vi "S-Curve Newton Method Time.vi"(4 "v_f":dbl, 6 "v_i":dbl, 7 "err":dbl, 8 "g":dbl, 9 "j":dbl, 10 "a":dbl, 11 "v":dbl) -> (3 "t_out":dbl)   [LabVIEW 2025]
uses:
  <vilib>/ptbypt/NI_PtbyPt.lvlib
panel:
  out "iterations":i32
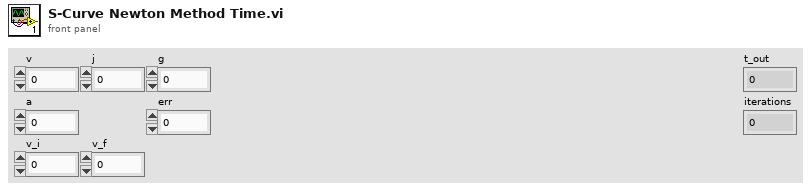
[diagram p1: front panel]
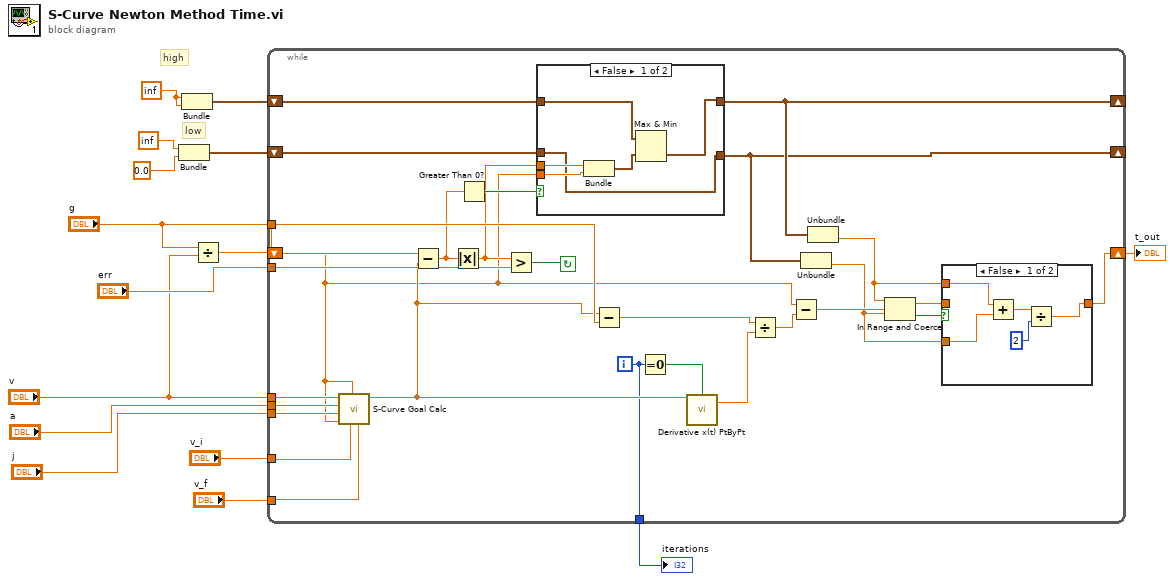
[diagram p0: block diagram]
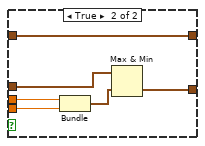
[diagram p2: hidden frame]
diagram:
  w6 = inf
  # "low"
  # "high"
  n1 = Bundle(inf, 0.0) -> (w2:cluster{dbl, dbl})  [unwired: 1 in]
  n2 = Bundle(w6, w6) -> (w5:cluster{dbl, dbl})  [unwired: 1 in]
  n3 = Divide(x="g", y="v") -> (x/y=w7:dbl)
  n4 = while {
    tunnel: "v" -> [w31]
    tunnel: "a" -> [w43]
    tunnel: "j" -> [w42]
    tunnel: "v_i" -> [w41]
    tunnel: "v_f" -> [w40]
    shift-right: [w19] -> w10
    shift-left: w7 -> [w16]
    tunnel: "g" -> [w36]
    tunnel: "err" -> [w39]
    shift-right: [w24] -> _
    shift-left: w5 -> [w25]
    shift-right: [w23] -> _
    shift-left: w2 -> [w27]
    tunnel: [w22] -> w1
    i -> [w22]
    stop <- w38 continue-if-true
    n5 = call "S-Curve Goal Calc.vi"("v_f"=w40, "v_i"=w41, "x"=w16, "t"=w16, "j"=w42, "a"=w43, "v"=w31) -> ("goal"=w33:dbl)  [unwired: 4 in]
    n6 = Subtract(x=w36, y=w33) -> (x-y=w29:dbl)
    n7 = Absolute Value(x=w29) -> (abs(x)=w26:dbl)
    n8 = Greater Than 0?(x=w29) -> (x > 0?=w28:bool)
    n9 = Greater?(x=w26, y=w39) -> (0:w38:bool)
    n10 = case shown="False" w28 {
      tunnel: w27 -> [w44 w52]
      tunnel: w26 -> [w48 w55]
      tunnel: w16 -> [w47 w54]
      tunnel: [w44 w51] -> w23
      tunnel: w25 -> [w46 w50]
      tunnel: [w45 w50] -> w24
      frame False {
        n11 = Bundle(w48, w47) -> (w49:cluster{dbl, dbl})  [unwired: 1 in]
        n12 = Max & Min(x=w46, y=w49) -> (min(x,y)=w45:cluster{dbl, dbl})  [unwired: 1 out]
      }
      frame True {
        n13 = Bundle(w55, w54) -> (w53:cluster{dbl, dbl})  [unwired: 1 in]
        n14 = Max & Min(x=w52, y=w53) -> (min(x,y)=w51:cluster{dbl, dbl})  [unwired: 1 out]
      }
    }
    n15 = Subtract(x=w33, y=w36) -> (x-y=w35:dbl)
    n16 = Equal To 0?(x=w22) -> (x = 0?=w30:bool)
    n17 = call <vilib>:"Derivative x(t) PtByPt.vi"("initialize"=w30, "x"=w33) -> ("dx/dt"=w32:dbl)  [unwired: 2 in, 1 out]
    n18 = Divide(x=w35, y=w32) -> (x/y=w37:dbl)
    n19 = Subtract(x=w16, y=w37) -> (x-y=w34:dbl)
    n20 = Unbundle(w23) -> (w17:dbl)  [unwired: 1 out]
    n21 = Unbundle(w24) -> (w18:dbl)  [unwired: 1 out]
    n22 = In Range and Coerce(upper limit=w18, x=w34, lower limit=w17) -> (coerced(x)=w20:dbl, In Range?=w21:bool)
    n23 = case shown="False" w21 {
      tunnel: w20 -> [_ w61]
      tunnel: [w56 w61] -> w19
      tunnel: w18 -> [w60 _]
      tunnel: w17 -> [w59 _]
      frame False {
        n24 = Add(x=w60, y=w59) -> (x+y=w58:dbl)
        n25 = Divide(x=w58, y=2) -> (x/y=w56:dbl)
      }
      frame True {
      }
    }
  }
  "t_out" <- w10
  "iterations" <- w1
